vi "Report.vi"(8 "error in (no error)":errorcluster) -> (0 "error out":errorcluster)   [LabVIEW 2018]
uses:
  Global_Variable/A131258.vi
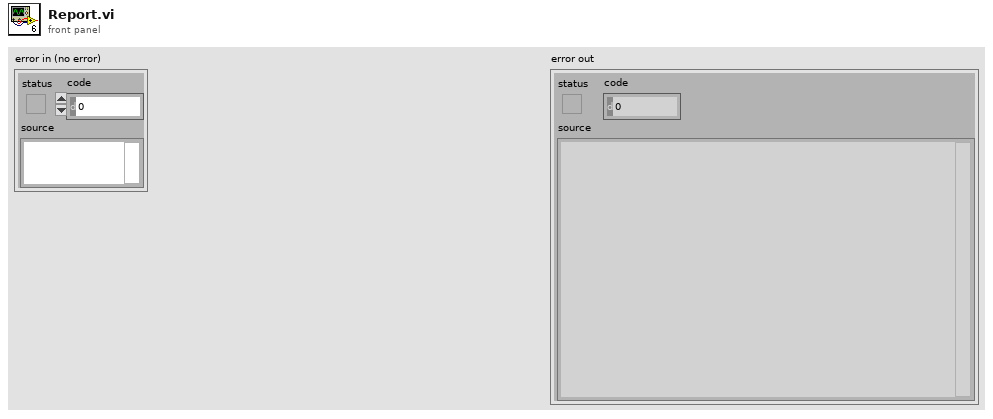
[diagram p1: front panel]
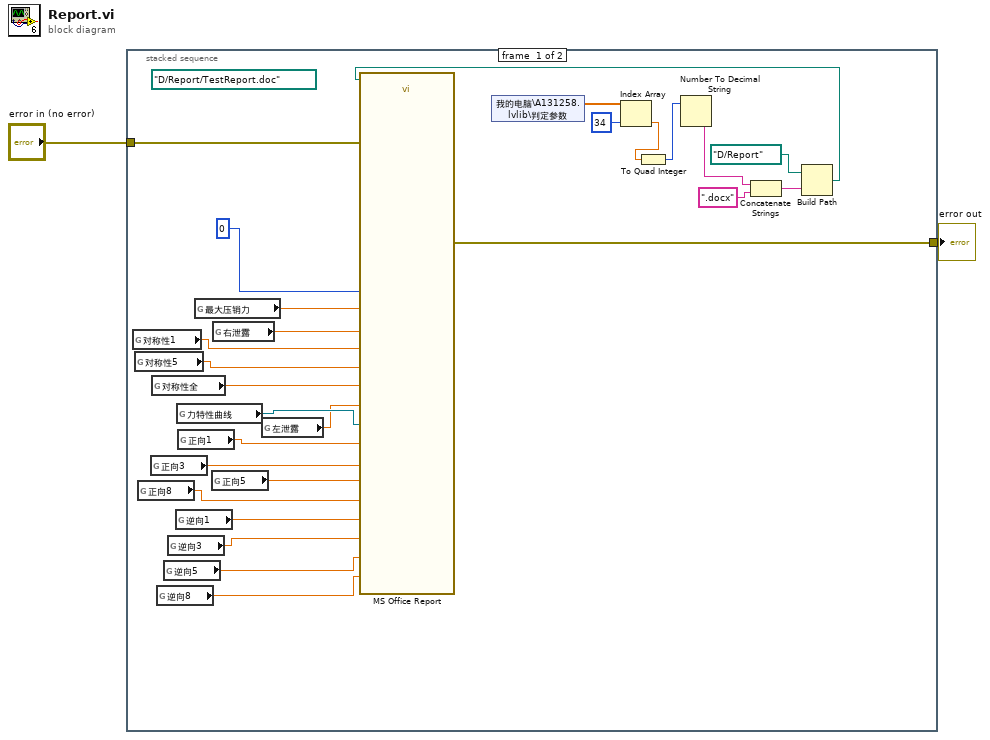
[diagram p0: block diagram]
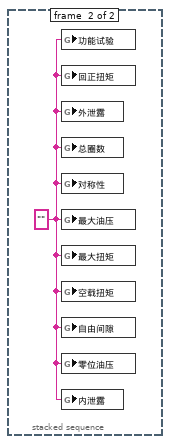
[diagram p2: hidden frame]
diagram:
  n1 = stacked-sequence {
    tunnel: [w29 _] -> w2
    tunnel: "error in (no error)" -> [w28 _]
    frame #0 {
      (unwired) path "D:/Report/TestReport.doc" ("Path to Save Report")
      n2 = global read "A131258.vi" "对称性1"() -> (w23:dbl)
      n3 = global read "A131258.vi" "对称性5"() -> (w22:dbl)
      n4 = global read "A131258.vi" "正向8"() -> (w16:dbl)
      n5 = global read "A131258.vi" "正向3"() -> (w18:dbl)
      n6 = global read "A131258.vi" "对称性全"() -> (w21:dbl)
      n7 = global read "A131258.vi" "逆向8"() -> (w12:dbl)
      n8 = global read "A131258.vi" "逆向5"() -> (w13:dbl)
      n9 = global read "A131258.vi" "逆向3"() -> (w14:dbl)
      n10 = global read "A131258.vi" "逆向1"() -> (w15:dbl)
      n11 = global read "A131258.vi" "力特性曲线"() -> (w26:refnum<vi>)
      n12 = global read "A131258.vi" "正向1"() -> (w20:dbl)
      n13 = global read "A131258.vi" "最大压销力"() -> (w25:dbl)
      n14 = global read "A131258.vi" "正向5"() -> (w17:dbl)
      n15 = global read "A131258.vi" "右泄露"() -> (w24:dbl)
      n16 = global read "A131258.vi" "左泄露"() -> (w19:dbl)
      n17 = shared-variable "我的电脑\\A131258.lvlib\\判定参数"() -> (w8:sgl[])  [unwired: 1 in, 1 out]
      n18 = Index Array(array=w8, index=34 ("索引")) -> (element=w3:sgl)
      n19 = To Quad Integer(1:w3) -> (0:w4:i64)
      n20 = Number To Decimal String(number=w4) -> (decimal integer string=w6:string)  [unwired: 1 in]
      n21 = Concatenate Strings(w6, ".docx" ("字符串")) -> (w11:string)
      n22 = Build Path(base path=path "D:/Report" ("基路径"), name or relative path=w11) -> (appended path=w5:path)
      n23 = call "MS Office Report"("Path to Save Report"=w5, "产品型号"=0, "压销力"=w25, "右泄露"=w24, "对称性1mpa"=w23, "对称性5mpa"=w22, "error in (no error)"=w28, "对称性全部"=w21, "左泄露"=w19, "曲线"=w26, "正向1"=w20, "正向3"=w18, "正向5"=w17, "正向8"=w16, "逆向1"=w15, "逆向3"=w14, "逆向5"=w13, "逆向8"=w12) -> ("error out"=w29:errorcluster)  [unwired: 8 in, 1 out]
    }
    frame #1 {
      w30 = "" ("内泄露")
      n24 = global write "检测结果.vi" "功能试验"(w30) -> ()
      n25 = global write "检测结果.vi" "回正扭矩"(w30) -> ()
      n26 = global write "检测结果.vi" "外泄露"(w30) -> ()
      n27 = global write "检测结果.vi" "总圈数"(w30) -> ()
      n28 = global write "检测结果.vi" "对称性"(w30) -> ()
      n29 = global write "检测结果.vi" "最大油压"(w30) -> ()
      n30 = global write "检测结果.vi" "最大扭矩"(w30) -> ()
      n31 = global write "检测结果.vi" "空载扭矩"(w30) -> ()
      n32 = global write "检测结果.vi" "自由间隙"(w30) -> ()
      n33 = global write "检测结果.vi" "零位油压"(w30) -> ()
      n34 = global write "检测结果.vi" "内泄露"(w30) -> ()
    }
  }
  "error out" <- w2
